vi "CalcDelayTime.vi"(9 "Uncertainties":dbl[][](array[numeric]), 10 "StepType":string, 11 "Step Data":dbl[][][](array[numeric])) -> (3 "DelayTime Range":dbl[][][](array[numeric]))   [LabVIEW 2014]
uses:
  <vilib>/Analysis/NI_AALBase.lvlib
panel:
  out "Waveform Graph":cluster{"Numeric":dbl, dbl, dbl[]}(graph)
  # "DT + Unc"
  # "Delay Time"
  # "DT - Unc"
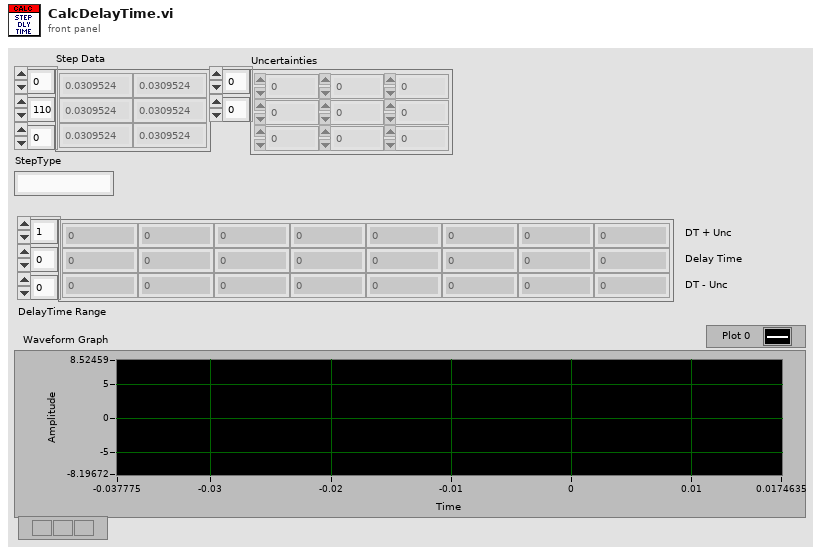
[diagram p1: front panel]
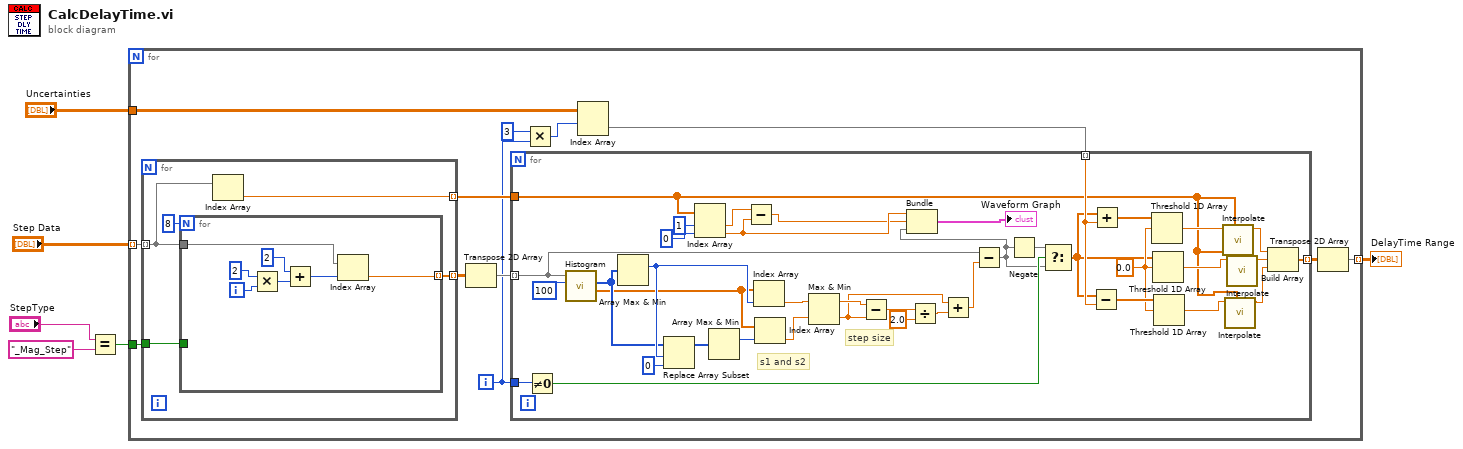
[diagram p0: block diagram]
diagram:
  n1 = Equal?(x="StepType", y="_Mag_Step") -> (x = y?=w3:bool)
  n2 = for {
    tunnel: "Step Data" -> [w18] mode=indexing
    tunnel: w3 -> [w17]
    tunnel: [w7] -> w2 mode=indexing
    tunnel: "Uncertainties" -> [w10]
    i -> [w12]
    n3 = for {
      tunnel: w18 -> [w59] mode=indexing
      tunnel: [w62] -> w16 mode=indexing
      tunnel: w17 -> [w61]
      tunnel: [w58] -> w14 mode=indexing
      n4 = for {
        N: 8 -> [_]
        tunnel: w59 -> [w64]
        tunnel: [w63] -> w62 mode=indexing
        tunnel: w61 -> [_]
        i -> [w69]
        n5 = Multiply(x=2, y=w69) -> (x*y=w67:i32)
        n6 = Add(x=2, y=w67) -> (x+y=w65:i32)
        n7 = Index Array(array=w64, index=w65) -> (element=w63:dbl)
      }
      n8 = Index Array(array=w59) -> (element=w58:dbl)  [unwired: 1 in]
    }
    n9 = Transpose 2D Array(2D array=w16) -> (transposed array=w15:dbl[][])
    n10 = Multiply(x=3, y=w12) -> (x*y=w9:i32)
    n11 = Index Array(array=w10, index (row)=w9) -> (element=w8:dbl[])  [unwired: 1 in]
    n12 = for {
      tunnel: w15 -> [w46] mode=indexing
      tunnel: w14 -> [w27]
      tunnel: w12 -> [w42]
      tunnel: [w34] -> w13 mode=indexing
      tunnel: w8 -> [w38] mode=indexing
      w35 = 0.0 ("threshold y")
      # "step size"
      # "s1 and s2"
      n13 = Not Equal To 0?(x=w42) -> (x != 0?=w40:bool)
      n14 = call <vilib>:"Histogram.vi"("intervals"=100, "X"=w46) -> ("X Values"=w50:dbl[], "Histogram: h(x)"=w51:i32[])  [unwired: 6 in, 2 out]
      n15 = Array Max & Min(array=w51) -> (max index (indices)=w52:i32)  [unwired: 3 out]
      n16 = Replace Array Subset(array=w51, new element=0 ("new element/subarray"), index=w52) -> (w54:i32[])
      n17 = Index Array(array=w27, index #1=1 ("index"), index #2=0 ("index")) -> (element #1=w24:dbl, element #2=w21:dbl)
      n18 = Array Max & Min(array=w54) -> (max index (indices)=w55:i32)  [unwired: 3 out]
      n19 = Subtract(x=w24, y=w21) -> (x-y=w20:dbl)
      n20 = Index Array(array=w50, index=w52) -> (element=w56:dbl)
      n21 = Index Array(array=w50, index=w55) -> (element=w44:dbl)
      n22 = Max & Min(x=w56, y=w44) -> (max(x,y)=w57:dbl, min(x,y)=w39:dbl)
      n23 = Subtract(x=w57, y=w39) -> (x-y=w48:dbl)
      n24 = Divide(x=w48, y=2.0) -> (x/y=w45:dbl)
      n25 = Add(x=w39, y=w45) -> (x+y=w43:dbl)
      n26 = Subtract(x=w46, y=w43) -> (x-y=w19:dbl[])
      n27 = Bundle("Numeric"=w21, w20, w19) -> (→"Waveform Graph":cluster{"Numeric":dbl, dbl, dbl[]})  [unwired: 1 in]
      n28 = Negate(x=w19) -> (-x=w41:dbl[])
      n29 = Select(t=w41, s=w40, f=w19) -> (s? t:f=w23:dbl[])
      n30 = Subtract(x=w23, y=w38) -> (x-y=w36:dbl[])
      n31 = Add(x=w23, y=w38) -> (x+y=w37:dbl[])
      n32 = Threshold 1D Array(2:w35, 3:w37) -> (0:w30:dbl)  [unwired: 1 in]
      n33 = Threshold 1D Array(2:w35, 3:w23) -> (0:w29:dbl)  [unwired: 1 in]
      n34 = Threshold 1D Array(2:w35, 3:w36) -> (0:w28:dbl)  [unwired: 1 in]
      n35 = call "Interpolate.vi"("Array"=w27, "Index"=w30) -> ("Value"=w33:dbl)  [unwired: 9 in]
      n36 = call "Interpolate.vi"("Array"=w27, "Index"=w28) -> ("Value"=w31:dbl)  [unwired: 9 in]
      n37 = call "Interpolate.vi"("Array"=w27, "Index"=w29) -> ("Value"=w32:dbl)  [unwired: 9 in]
      n38 = Build Array(w33, w32, w31) -> (w34:dbl[])
    }
    n39 = Transpose 2D Array(2D array=w13) -> (transposed array=w7:dbl[][])
  }
  "DelayTime Range" <- w2
